vi "Operation Number.vi"(8 "error in (no error)":errorcluster, 11 "Client Message in":refnum<class "Client Message.lvclass">) -> (0 "error out":errorcluster, 2 "Operation Num":i32, 3 "Client Message out":refnum<class "Client Message.lvclass">)   [LabVIEW 2022 SP3, in "obs-websocket-lv.lvlib" / "Client Message.lvclass"]
uses:
  Client Message.lvclass
  Client Message.lvclass/Client Message.ctl
  obs-websocket-lv.lvlib
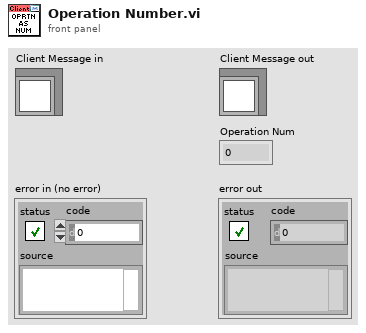
[diagram p1: front panel]
types:
  T1 = typedef "obs-websocket-lv.lvlib/Client Operation.ctl" = enum16{"Identify", "Reidentify", "Request", "RequestBatch"}
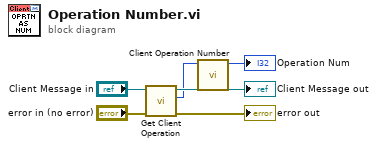
[diagram p0: block diagram]
diagram:
  n1 = call-dynamic "Get Client Operation.vi"("error in (no error)"="error in (no error)", "Client Message in"="Client Message in") -> ("error out"=→"error out":errorcluster, "Client Operation"=w2:T1, "Client Message out"=→"Client Message out":refnum<class "Client Message.lvclass">)  [unwired: 7 in]
  n2 = call "Client Operation Number.vi"("Client Operation"=w2) -> ("Op"=→"Operation Num":i32)  [unwired: 10 in]
